vi "提取IOTdata.vi"() -> (3 "IOT DATA":string[](array[string]))   [LabVIEW 2017]
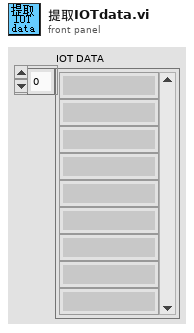
[diagram p1: front panel]
types:
  T1 = typedef "IOT time.ctl" = cluster{"Work":string, "Inflow":string, "Outflow":string, "Wait":string}
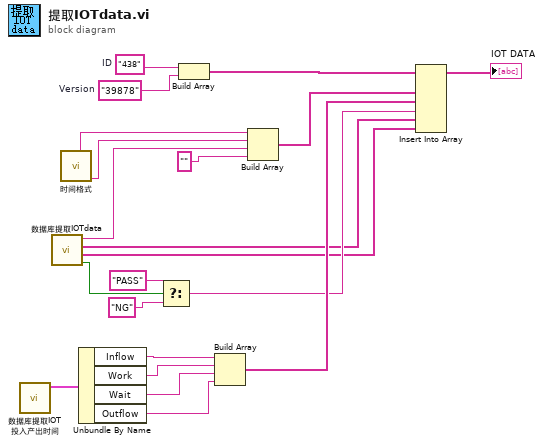
[diagram p0: block diagram]
diagram:
  w4 = "39878"  # Version
  w5 = "438"  # ID
  n1 = call "数据库提取IOT 投入产出时间.vi"() -> ("IOT time"=w17:T1)  [unwired: 11 in]
  n2 = call "数据库提取IOTdata.vi"() -> ("in spec?"=w10:bool, "data"=w1:string[], "次数&压力"=w2:string[], "SN"=w19:string)  [unwired: 8 in]
  n3 = call "时间格式.vi"() -> ("Time"=w20:string, "Date"=w21:string)  [unwired: 7 in, 3 out]
  n4 = Unbundle By Name(w17) -> ("Inflow"=w16:string, "Work"=w15:string, "Wait"=w14:string, "Outflow"=w13:string)
  n5 = Select(t="PASS", s=w10, f="NG") -> (s? t:f=w7:string)
  n6 = Build Array(w5, w4) -> (w3:string[])
  n7 = Build Array(w16, w15, w14, w13) -> (w11:string[])
  n8 = Build Array(w21, w20, w19, "") -> (w12:string[])
  n9 = Insert Into Array(array=w3, new element #1=w12, new element #2=w11, new element #3=w7, new element #4=w2, new element #5=w1) -> (→"IOT DATA":string[])  [unwired: 1 in]
